vi "模拟输入_有限(可重触发).vi"() -> ()   [LabVIEW 2013]
doc: "This example demonstrates how to acquire a finite amount of data."
uses:
  <userlib>/ArtDAQ/_SubVI/ArtDAQ_CreateAIVoltageChan.vi
  <userlib>/ArtDAQ/_SubVI/ArtDAQ_CfgSampClkTiming.vi
  <userlib>/ArtDAQ/_SubVI/ArtDAQ_CfgDigEdgeStartTrig.vi
  <userlib>/ArtDAQ/_SubVI/ArtDAQ_Read Analog DBL NChan NSamp.vi
panel:
  in  "触发源":string="/Dev1/PFI1"
  in  "触发边沿":i32(ring)=10280 items=["上升"=10280, "下降"=10171]
  in  "可重?":bool=TRUE
  in  "Stop":bool
  out "波形图":dbl[][](graph)
  in  "采样速率":dbl=10000.0 format="%#_13g"
  in  "每通道采样点数":i32=1000
  in  "接线端配置":i32(ring)=10083 items=["默认"=-1, "单端"=10083, "非参考单端"=10078, "差分"=10106, "伪差分"=12529]
  in  "最小值(V)":dbl=-10.0 format="%#_13g"
  in  "最大值(V)":dbl=10.0 format="%#_13g"
  in  "物理通道":string(combo)="Dev1/ai0"
  out "错误":errorcluster
  # "通道属性"
  # "定时"
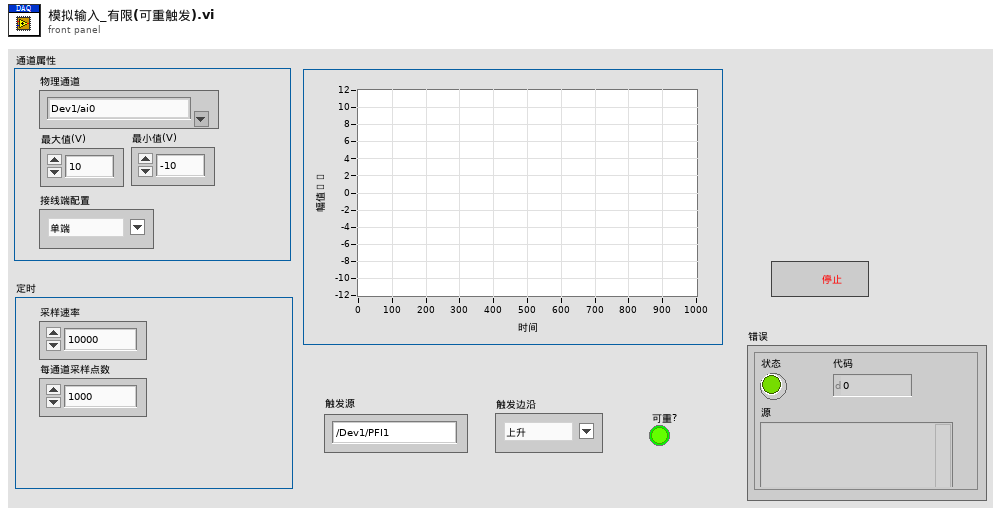
[diagram p1: front panel]
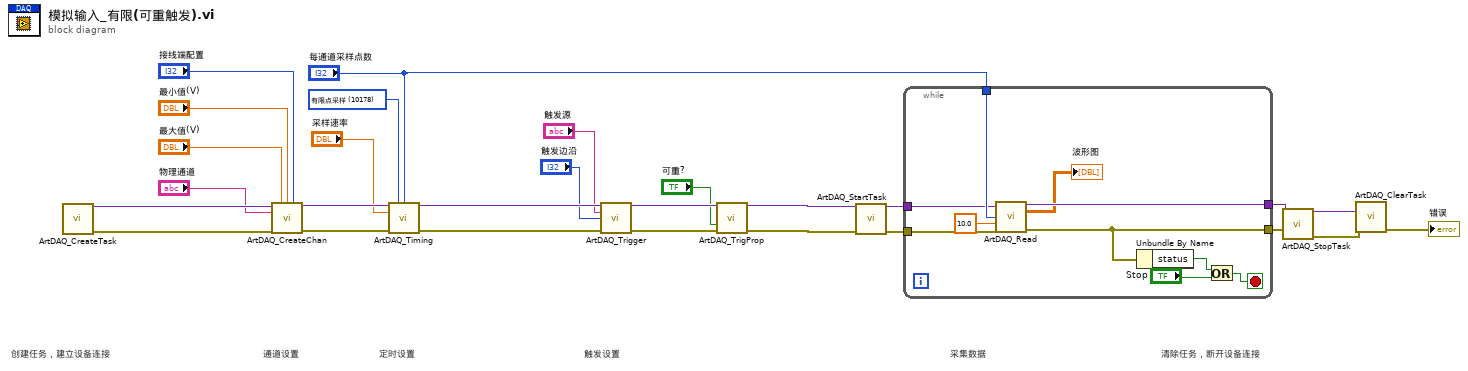
[diagram p0: block diagram]
diagram:
  w21 = 10178 items=["有限点采样"=10178, "连续采样"=10123] ("SampleMode")
  # "清除任务，断开设备连接"
  # "采集数据"
  # "触发设置"
  # "定时设置"
  # "通道设置"
  # "创建任务，建立设备连接"
  n1 = call <userlib>:"ArtDAQ_CreateTask.vi"() -> ("任务句柄"=w17:variant, "错误输出"=w27:errorcluster)  [unwired: 14 in]
  n2 = call-poly <userlib>:"ArtDAQ_CreateChan.vi"("任务句柄"=w17, "最大值"="最大值(V)", "最小值"="最小值(V)", "接线端配置"="接线端配置", "物理通道"="物理通道", "错误输入"=w27) -> ("任务句柄"=w23:variant, "错误输出"=w22:errorcluster)  [unwired: 8 in]
  n3 = call-poly <userlib>:"ArtDAQ_Timing.vi"("任务句柄"=w23, "采样模式"=w21, "每通道采样数"="每通道采样点数", "采样率"="采样速率", "错误输入"=w22) -> ("任务句柄"=w14:variant, "错误输出"=w12:errorcluster)  [unwired: 9 in]
  n4 = call-poly <userlib>:"ArtDAQ_Trigger.vi"("任务句柄"=w14, "触发源"="触发源", "边沿"="触发边沿", "错误输入"=w12) -> ("任务句柄"=w3:variant, "错误输出"=w2:errorcluster)  [unwired: 10 in]
  n5 = call-poly <userlib>:"ArtDAQ_TrigProp.vi"("任务句柄"=w3, "可重?"="可重?", "错误输入"=w2) -> ("任务句柄"=w13:variant, "错误输出"=w11:errorcluster)  [unwired: 11 in]
  n6 = call <userlib>:"ArtDAQ_StartTask.vi"("任务句柄"=w13, "错误输入"=w11) -> ("任务句柄"=w9:variant, "错误输出"=w8:errorcluster)  [unwired: 12 in]
  n7 = while {
    tunnel: "每通道采样点数" -> [w37]
    tunnel: w9 -> [w36]
    tunnel: w8 -> [w35]
    tunnel: [w34] -> w7
    tunnel: [w29] -> w6
    stop <- w28 stop-if-true
    n8 = call-poly <userlib>:"ArtDAQ_Read.vi"("任务句柄"=w36, "每通道采样数"=w37, "超时s"=10.0 ("Timeout"), "错误输入"=w35) -> ("任务句柄"=w34:variant, "数据"=→"波形图":dbl[][], "错误输出"=w29:errorcluster)  [unwired: 8 in, 1 out]
    n9 = Unbundle By Name(w29) -> ("status"=w31:bool)
    n10 = Or(x=w31, y="Stop") -> (x .or. y?=w28:bool)
  }
  n11 = call <userlib>:"ArtDAQ_StopTask.vi"("任务句柄"=w7, "错误输入"=w6) -> ("任务句柄"=w16:variant, "错误输出"=w15:errorcluster)  [unwired: 12 in]
  n12 = call <userlib>:"ArtDAQ_ClearTask.vi"("任务句柄"=w16, "错误输入"=w15) -> ("错误输出"=→"错误":errorcluster)  [unwired: 13 in]
